vi "SetGain.vi"(8 "error in":errorcluster, 10 "Gain":enum16{"Low", "High"}(ring), 11 "camera.nit in":refnum<class "camera.lvclass">) -> (0 "error out":errorcluster)   [LabVIEW 2020, in "camera.lvclass"]
uses:
  camera.lvclass
  079f7f5f-754c-4484-b792-9b60d2a2114c.vi
  camera.lvclass/camera.ctl
  lib/O-PL.dll
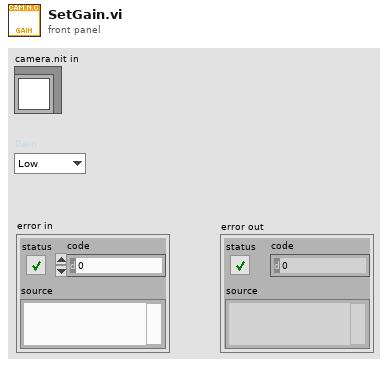
[diagram p1: front panel]
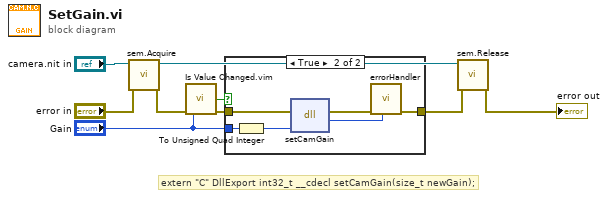
[diagram p0: block diagram]
diagram:
  # "extern \"C\" DllExport int32_t __cdecl setCamGain(size_t newGain);"
  n1 = call "sem.Acquire.vi"("error in"="error in", "camera.nit in"="camera.nit in") -> ("error out"=w3:errorcluster)  [unwired: 9 in]
  n2 = call "Is Value Changed.vim"("value"="Gain") -> ("changed or first call?"=w7:bool)
  n3 = case shown="True" w7 {
    tunnel: "Gain" -> [_ w13]
    tunnel: w3 -> [w8 w14]
    tunnel: [w8 w9] -> w2
    frame False {
    }
    frame True {
      n4 = To Unsigned Quad Integer(1:w13) -> (0:w12:u64)
      n5 = dll-call lib="C:/Users/pittsburger.SOLARIS/Desktop/v0.8/lib/O-PL.dll" fn="setCamGain"(error in=w14, "gain"=w12) -> (error out=w11:errorcluster, "return type"=w10:i32)  [unwired: 3 in, 1 out]
      n6 = call "errorHandler.vi"("code"=w10, "error in"=w11) -> ("error out"=w9:errorcluster)  [unwired: 9 in]
    }
  }
  n7 = call "sem.Release.vi"("error in"=w2, "camera.nit in"="camera.nit in") -> ("error out"=→"error out":errorcluster)  [unwired: 9 in]
